vi "Viasala Simulated Data.vi"(8 "error in (no error)":errorcluster) -> (0 "error out":errorcluster, 3 "Viasala Data Output":T1)   [LabVIEW 2023]
uses:
  Drivers/Viasala Indigo 520/Type Definitions/Viasala Indigo 520 Data.ctl
  <vilib>/numeric/Random Number (Range) DBL.vi
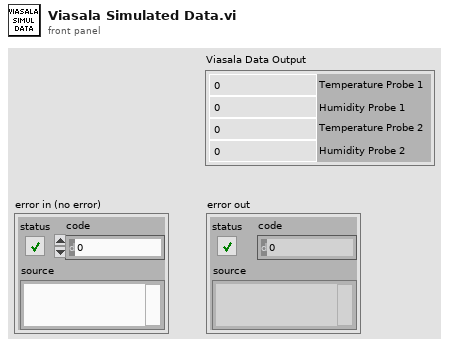
[diagram p1: front panel]
types:
  T1 = typedef "Viasala Indigo 520 Data.ctl" = cluster{"Temperature Probe 1":dbl, "Humidity Probe 1":dbl, "Temperature Probe 2":dbl, "Humidity Probe 2":dbl}
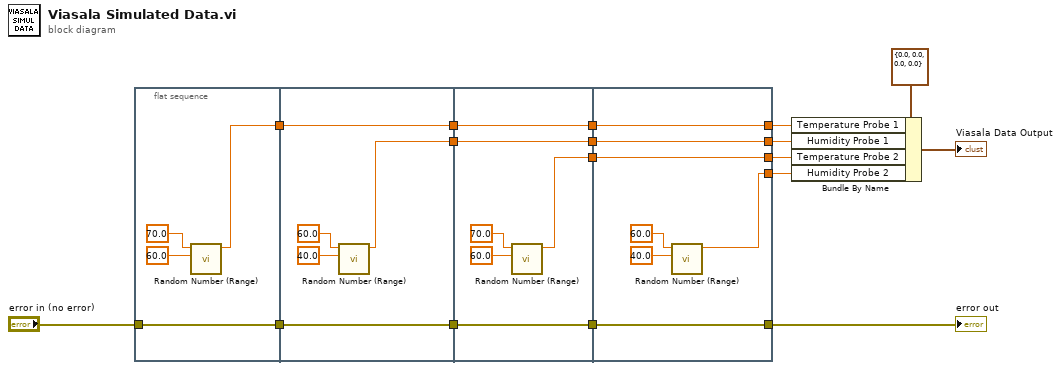
[diagram p0: block diagram]
diagram:
  n1 = flat-sequence {
    tunnel: "error in (no error)" -> [w19]
    tunnel: [w19] -> w17
    tunnel: [w18] -> w13
    tunnel: w17 -> [w26]
    tunnel: [w26] -> w16
    tunnel: w13 -> [w23]
    tunnel: [w23] -> w12
    tunnel: [w22] -> w10
    tunnel: w16 -> [w32]
    tunnel: w12 -> [w29]
    tunnel: w10 -> [w28]
    tunnel: [w32] -> w5
    tunnel: [w29] -> w4
    tunnel: [w28] -> w3
    tunnel: [w27] -> w2
    tunnel: [w36] -> w8
    tunnel: [w37] -> w9
    tunnel: [w38] -> w11
    tunnel: [w39] -> w15
    tunnel: w5 -> [w39]
    tunnel: w4 -> [w38]
    tunnel: w3 -> [w37]
    tunnel: w2 -> [w36]
    tunnel: [w33] -> w1
    frame #0 {
      n2 = call-poly <vilib>:"Random Number (Range).vi"("lower bound (0)"=60.0, "upper bound (100)"=70.0) -> ("number"=w18:dbl)  [unwired: 9 in]
    }
    frame #1 {
      n3 = call-poly <vilib>:"Random Number (Range).vi"("lower bound (0)"=40.0, "upper bound (100)"=60.0) -> ("number"=w22:dbl)  [unwired: 9 in]
    }
    frame #2 {
      n4 = call-poly <vilib>:"Random Number (Range).vi"("lower bound (0)"=60.0, "upper bound (100)"=70.0) -> ("number"=w27:dbl)  [unwired: 9 in]
    }
    frame #3 {
      n5 = call-poly <vilib>:"Random Number (Range).vi"("lower bound (0)"=40.0, "upper bound (100)"=60.0) -> ("number"=w33:dbl)  [unwired: 9 in]
    }
  }
  n6 = Bundle By Name(cluster=T1 {"Temperature Probe 1"=0.0, "Humidity Probe 1"=0.0, "Temperature Probe 2"=0.0, "Humidity Probe 2"=0.0} ("Viasala Data Output"), "Temperature Probe 1"=w11, "Humidity Probe 1"=w9, "Temperature Probe 2"=w8, "Humidity Probe 2"=w1) -> (→"Viasala Data Output":T1)
  "error out" <- w15
